vi "Modify Data format to R2_filled+split.vi"(6 "Current set number in one current mode":i32=48, 7 "Scan number":i32=10, 8 "modified error":errorcluster, 9 "modified Data path":path, 10 "original error":errorcluster, 11 "original Data path":path) -> ()   [LabVIEW 2023]
uses:
  <vilib>/Utility/error.llb/DialogType.ctl
panel:
  out "floor(x/y)":i32
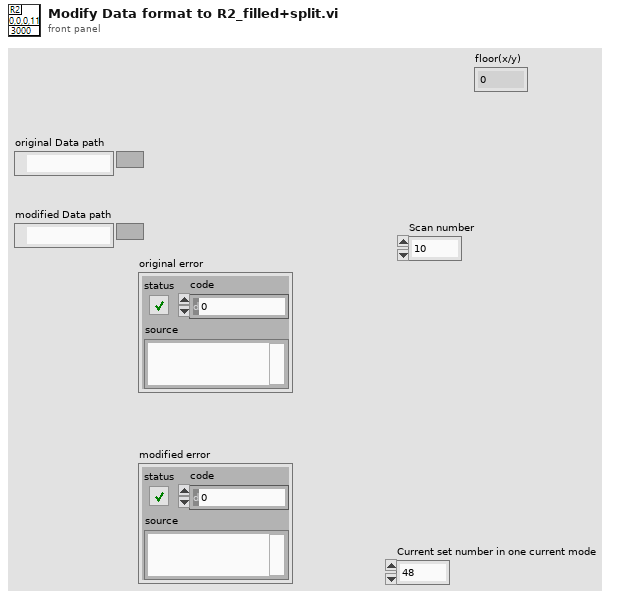
[diagram p1: front panel]
types:
  T1 = enum16{"open", "replace", "create", "open or create", "replace or create", "replace or create with confirmation"}
  T2 = typedef "DialogType.ctl" = u16
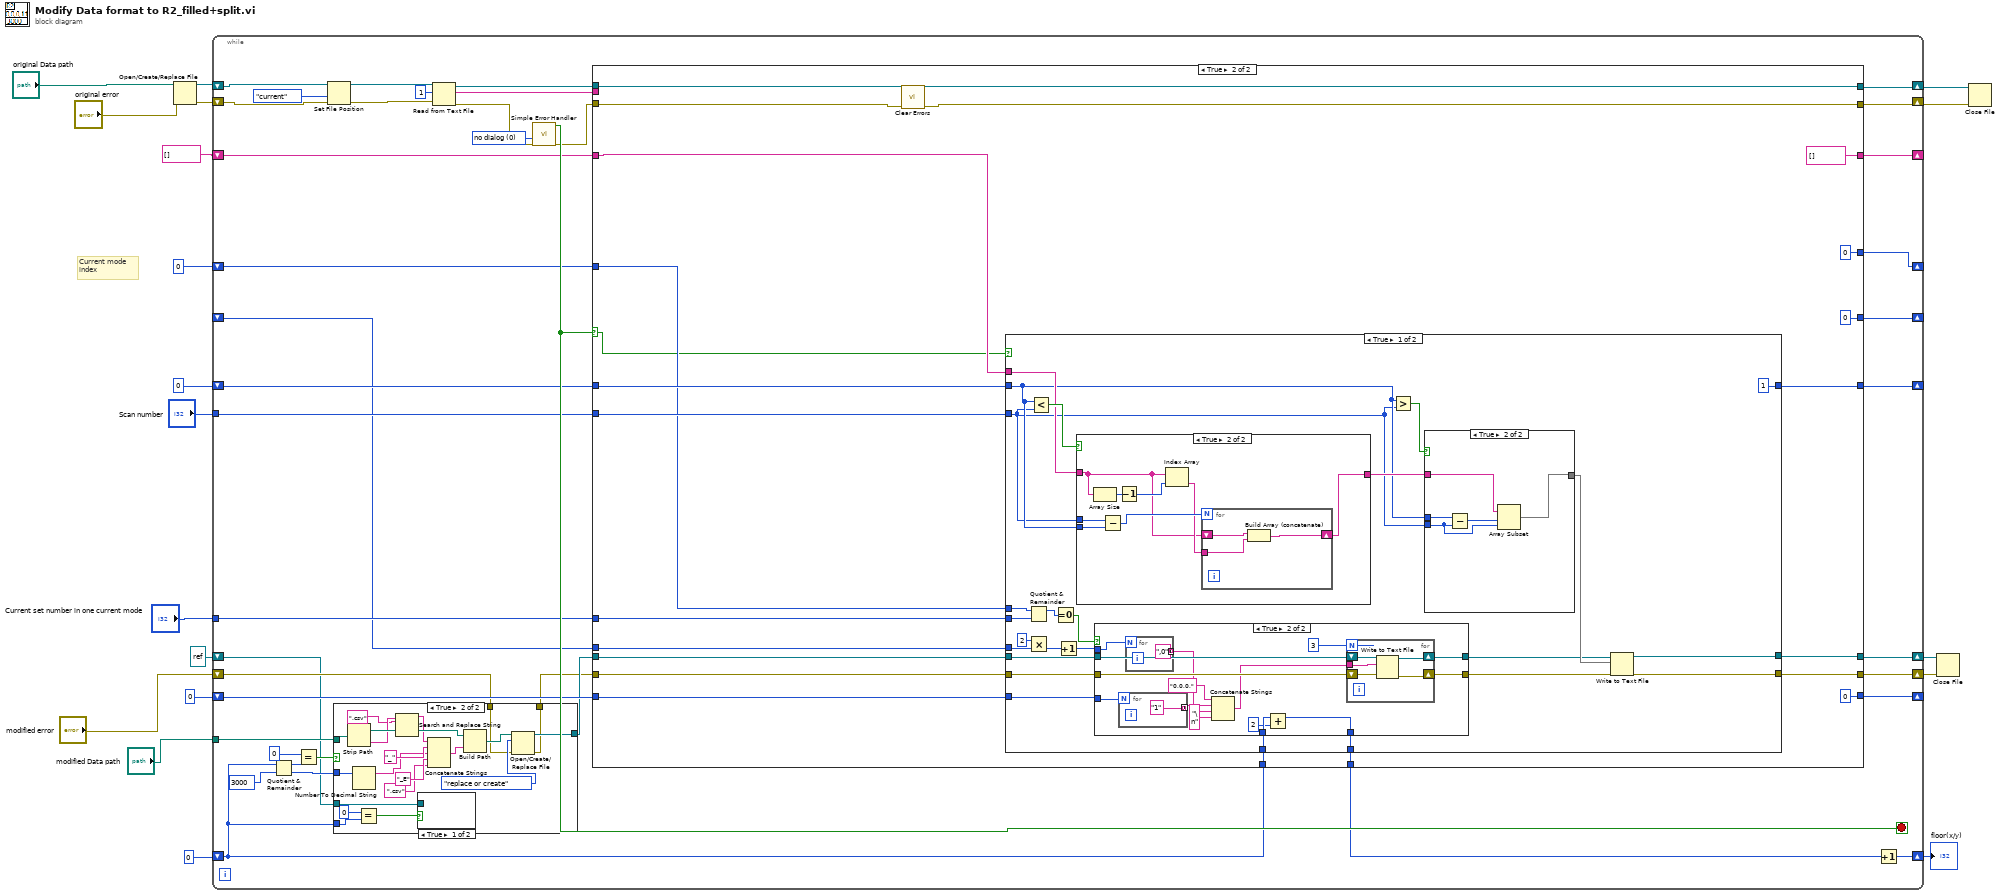
[diagram p0: block diagram]
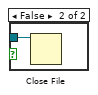
[diagram p3: hidden frame]
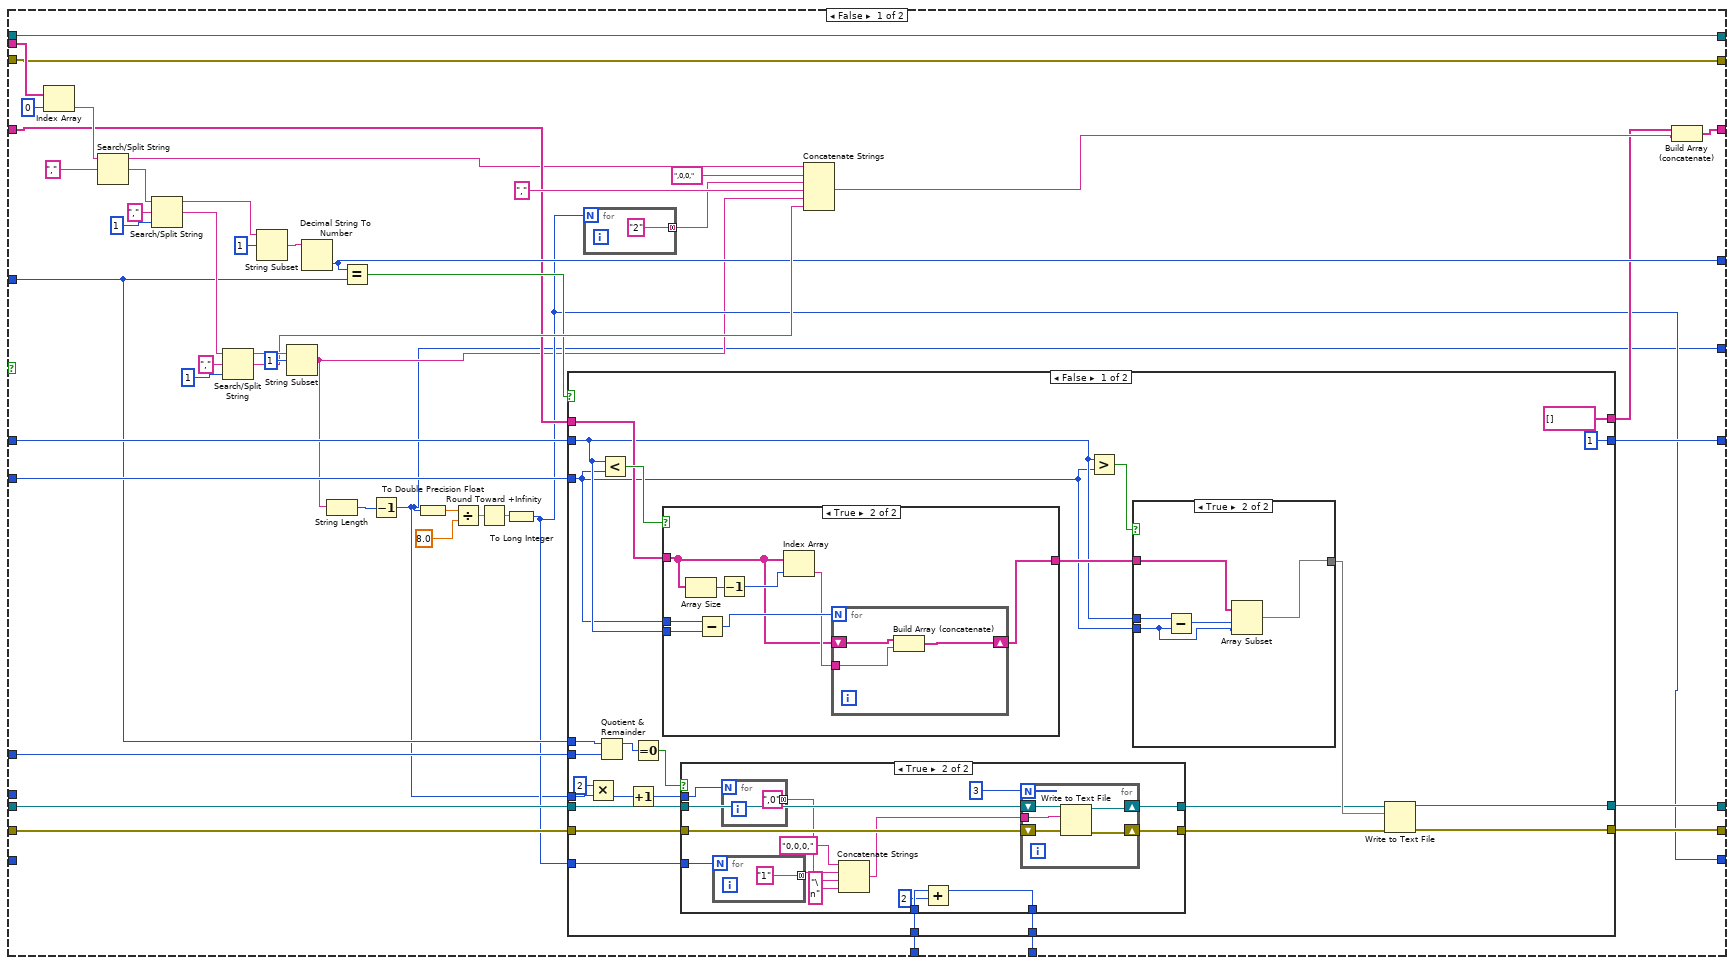
[diagram p4: hidden frame]
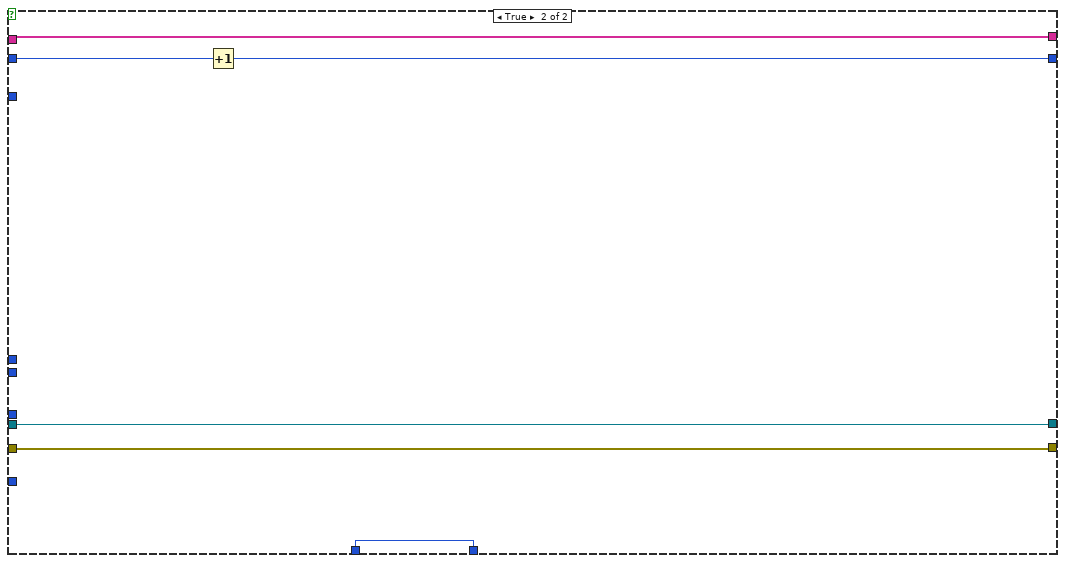
[diagram p8: hidden frame]
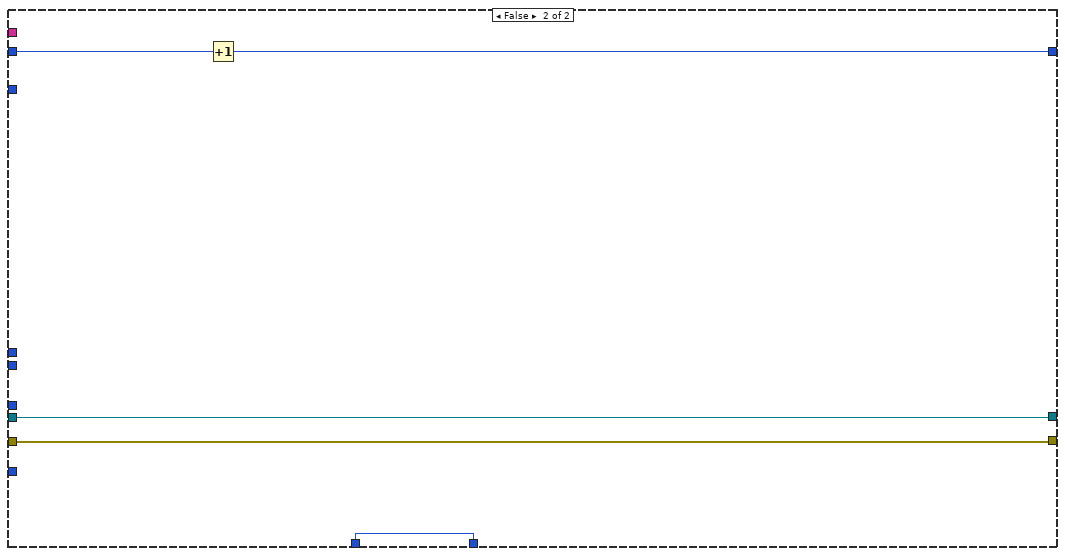
[diagram p12: hidden frame]
diagram:
  # "Current mode\nindex"
  n1 = Open/Create/Replace File(file path (use dialog)="original Data path", error in="original error") -> (refnum out=w17:refnum<file>, error out=w18:errorcluster)  [unwired: 4 in, 1 out]
  n2 = while {
    shift-right: [w52] -> w13
    shift-left: w18 -> [w59]
    shift-right: [w51] -> w19
    shift-left: w17 -> [w50]
    shift-right: [w47] -> w15
    shift-left: refnum<file> refnum ("refnum out") -> [w26]
    shift-right: [w46] -> w14
    shift-left: "modified error" -> [w29]
    shift-right: [w35] -> _
    shift-left: string[] [] ("element") -> [w44]
    shift-right: [w40] -> _
    shift-left: 0 ("number") -> [w43]
    shift-right: [w41] -> _
    shift-left: 0 ("number") -> [w42]
    tunnel: "Scan number" -> [w39]
    tunnel: "Current set number in one current mode" -> [w38]
    shift-right: [w37] -> _
    shift-left: 0 ("32bit integer") -> [w36]
    tunnel: "modified Data path" -> [w27]
    shift-right: [w25] -> w1
    shift-left: 0 ("floor(x/y)") -> [w24]
    shift-right: [w22] -> _
    shift-left: _ -> [w21]
    stop <- w56 stop-if-true
    w57 = T2 0 items=["no dialog", "OK message", "continue or stop message", "OK message + warnings", "continue/stop + warnings"] ("type of dialog (OK msg:1)")
    n3 = Quotient & Remainder(x=w24, y=3000) -> (x-y*floor(x/y)=w34:i32, floor(x/y)=w31:i32)
    n4 = Equal?(x=0, y=w34) -> (x = y?=w32:bool)
    n5 = Set File Position(refnum=w50, from (0:start)=enum16{"start", "end", "current"}."current", error in=w59) -> (refnum out=w49:refnum<file>, error out=w48:errorcluster)  [unwired: 1 in]
    n6 = case shown="True" w32 {
      tunnel: w27 -> [_ w76]
      tunnel: w31 -> [_ w78]
      tunnel: [w61 w73] -> w30
      tunnel: w29 -> [w62 w72]
      tunnel: [w62 w71] -> w28
      tunnel: w26 -> [w61 w70]
      tunnel: w24 -> [_ w68]
      frame False {
      }
      frame True {
        n7 = Strip Path(path=w76) -> (stripped path=w82:path, name=w64:string)
        n8 = Number To Decimal String(number=w78) -> (decimal integer string=w77:string)  [unwired: 1 in]
        n9 = Equal?(x=0, y=w68) -> (x = y?=w66:bool)
        n10 = Search and Replace String(input string=w64, search string=".csv") -> (result string=w65:string)  [unwired: 6 in, 3 out]
        n11 = case shown="True" w66 {
          tunnel: w70 -> [_ w83]
          frame True {
          }
          frame False {
            n12 = Close File(refnum=w83) -> ()  [unwired: 1 in, 2 out]
          }
        }
        n13 = Concatenate Strings(w65, "_" ("string"), w77, "_E" ("string"), ".csv" ("string")) -> (w81:string)
        n14 = Build Path(base path=w82, name or relative path=w81) -> (appended path=w74:path)
        n15 = Open/Create/Replace File(file path (use dialog)=w74, error in=w72, operation (0:open)=T1."replace or create") -> (refnum out=w73:refnum<file>, error out=w71:errorcluster)  [unwired: 3 in, 1 out]
      }
    }
    n16 = Read from Text File(file (use dialog)=w49, count=1, error in=w48) -> (refnum out=w54:refnum<file>, text=w55:string[], error out=w53:errorcluster)  [unwired: 1 in, 1 out]
    n17 = call <vilib>:"Simple Error Handler.vi"("type of dialog (OK msg:1)"=w57, "error in (no error)"=w53) -> ("error?"=w56:bool, "error out"=w45:errorcluster)  [unwired: 3 in, 3 out]
    n18 = case shown="True" w56 {
      selector: w56 -> [_ w215]
      tunnel: w55 -> [w125 _]
      tunnel: w54 -> [w123 w228]
      tunnel: w45 -> [w122 w217]
      tunnel: [w123 w228] -> w51
      tunnel: [w122 w216] -> w52
      tunnel: w30 -> [w103 w223]
      tunnel: w28 -> [w102 w222]
      tunnel: [w101 w221] -> w47
      tunnel: [w100 w220] -> w46
      tunnel: w44 -> [w105 w224]
      tunnel: w43 -> [w99 w219]
      tunnel: w42 -> [w110 w227]
      tunnel: [w109 w226] -> w41
      tunnel: [w108 0] -> w40
      tunnel: w39 -> [w106 w225]
      tunnel: w38 -> [w98 w218]
      tunnel: [w90 0] -> w37
      tunnel: w36 -> [_ w212]
      tunnel: [w89 string[] [] ("element")] -> w35
      tunnel: w24 -> [w86 w207]
      tunnel: [w85 w208] -> w23
      tunnel: [w84 0] -> w22
      tunnel: w21 -> [_ w209]
      frame False {
        n19 = Index Array(array=w125, index=0) -> (element=w121:string)
        n20 = Search/Split String(string=w121, search string/char (-)=",") -> (substring before match=w93:string, match + rest of string=w130:string)  [unwired: 1 in, 1 out]
        n21 = Search/Split String(string=w130, search string/char (-)=",", offset (0)=1) -> (substring before match=w113:string, match + rest of string=w118:string)  [unwired: 1 out]
        n22 = Search/Split String(string=w118, search string/char (-)=",", offset (0)=1) -> (substring before match=w117:string, match + rest of string=w115:string)  [unwired: 1 out]
        n23 = String Subset(string=w113, offset (0)=1) -> (substring=w112:string)  [unwired: 1 in]
        n24 = String Subset(string=w117, offset (0)=1) -> (substring=w88:string)  [unwired: 1 in]
        n25 = Decimal String To Number(string=w112) -> (number=w108:i32)  [unwired: 2 in, 1 out]
        n26 = String Length(string=w88) -> (length=w87:i32)
        n27 = Equal?(x=w108, y=w99) -> (x = y?=w111:bool)
        n28 = Decrement(x=w87) -> (x-1=w84:i32)
        n29 = To Double Precision Float(number=w84) -> (double precision float=w96:dbl)
        n30 = Divide(x=w96, y=8.0) -> (x/y=w97:dbl)
        n31 = Round Toward +Infinity(x=w97) -> (ceil(x): smallest int >= x=w94:dbl)
        n32 = To Long Integer(number=w94) -> (32bit integer=w90:i32)
        n33 = case shown="False" w111 {
          tunnel: [1 w205] -> w109
          tunnel: w110 -> [w151 w206]
          tunnel: w106 -> [w150 _]
          tunnel: w105 -> [w154 w204]
          tunnel: [string[] [] ("element") w204] -> w104
          tunnel: w103 -> [w142 w203]
          tunnel: w102 -> [w141 w202]
          tunnel: [w148 w203] -> w101
          tunnel: [w147 w202] -> w100
          tunnel: w99 -> [w146 _]
          tunnel: w98 -> [w145 _]
          tunnel: w90 -> [w138 _]
          tunnel: w84 -> [w137 _]
          tunnel: w86 -> [w133 w201]
          tunnel: [w132 w201] -> w85
          frame False {
            n34 = Multiply(x=2, y=w137) -> (x*y=w136:i32)
            n35 = Quotient & Remainder(x=w146, y=w145) -> (x-y*floor(x/y)=w144:i32)  [unwired: 1 out]
            n36 = Less?(x=w151, y=w150) -> (x < y?=w155:bool)
            n37 = Increment(x=w136) -> (x+1=w134:i32)
            n38 = Equal To 0?(x=w144) -> (x = 0?=w143:bool)
            n39 = case shown="True" w155 {
              tunnel: w154 -> [w189 w191]
              tunnel: w150 -> [_ w195]
              tunnel: w151 -> [_ w194]
              tunnel: [w189 w190] -> w152
              frame False {
              }
              frame True {
                n40 = Array Size(array=w191) -> (size(s)=w197:i32)
                n41 = Subtract(x=w195, y=w194) -> (x-y=w193:i32)
                n42 = Decrement(x=w197) -> (x-1=w196:i32)
                n43 = Index Array(array=w191, index=w196) -> (element=w192:string)
                n44 = for {
                  N: w193 -> [_]
                  tunnel: w192 -> [w198]
                  shift-right: [w199] -> w190
                  shift-left: w191 -> [w200]
                  n45 = Build Array (concatenate)(w200, w198) -> (w199:string[])
                }
              }
            }
            n46 = case shown="True" w143 {
              tunnel: w142 -> [w160 w172]
              tunnel: w141 -> [w159 w171]
              tunnel: [w160 w169] -> w140
              tunnel: [w159 w168] -> w139
              tunnel: w138 -> [_ w167]
              tunnel: w134 -> [_ w166]
              tunnel: w133 -> [w158 w163]
              tunnel: [w158 w162] -> w132
              frame False {
              }
              frame True {
                n47 = for {
                  N: w167 -> [_]
                  tunnel: ["1" ("search string/char (-)")] -> w174 mode=concatenating
                }
                n48 = for {
                  N: w166 -> [_]
                  tunnel: [",0" ("search string/char (-)")] -> w164 mode=concatenating
                }
                n49 = Concatenate Strings("0,0,0," ("string"), w174, w164, "\n" ("string")) -> (w170:string)
                n50 = Add(x=w163, y=2) -> (x+y=w162:i32)
                n51 = for {
                  N: 3 -> [_]
                  shift-right: [w179] -> w169
                  shift-left: w172 -> [w182]
                  tunnel: w170 -> [w180]
                  shift-right: [w178] -> w168
                  shift-left: w171 -> [w181]
                  n52 = Write to Text File(file (use dialog)=w182, text=w180, error in=w181) -> (refnum out=w179:refnum<file>, error out=w178:errorcluster)  [unwired: 1 in, 1 out]
                }
              }
            }
            n53 = Greater?(x=w151, y=w150) -> (0:w153:bool)
            n54 = case shown="True" w153 {
              tunnel: w152 -> [w183 w187]
              tunnel: w151 -> [_ w188]
              tunnel: w150 -> [_ w185]
              tunnel: [w183 w184] -> w149
              frame False {
              }
              frame True {
                n55 = Subtract(x=w188, y=w185) -> (x-y=w186:i32)
                n56 = Array Subset(array=w187, index=w186, length=w185) -> (w184:string[])
              }
            }
            n57 = Write to Text File(file (use dialog)=w140, text=w149, error in=w139) -> (refnum out=w148:refnum<file>, error out=w147:errorcluster)  [unwired: 1 in, 1 out]
          }
          frame True {
            n58 = Increment(x=w206) -> (x+1=w205:i32)
          }
        }
        n59 = for {
          N: w90 -> [_]
          tunnel: ["2" ("search string/char (-)")] -> w91 mode=concatenating
        }
        n60 = Concatenate Strings(w93, ",0,0," ("string"), w91, "," ("string"), w88, w115) -> (w107:string)
        n61 = Build Array (concatenate)(w104, w107) -> (w89:string[])
      }
      frame True {
        n62 = call <vilib>:"Clear Errors.vi"("error in (no error)"=w217) -> ("error out"=w216:errorcluster)  [unwired: 5 in, 1 out]
        n63 = case shown="True" w215 {
          tunnel: [1 w300] -> w226
          tunnel: w227 -> [w248 w301]
          tunnel: w225 -> [w247 _]
          tunnel: w224 -> [w251 _]
          tunnel: w223 -> [w236 w299]
          tunnel: w222 -> [w235 w298]
          tunnel: [w245 w299] -> w221
          tunnel: [w244 w298] -> w220
          tunnel: w219 -> [w243 _]
          tunnel: w218 -> [w242 _]
          tunnel: w212 -> [w234 _]
          tunnel: w209 -> [w231 _]
          tunnel: [w230 w297] -> w208
          tunnel: w207 -> [w229 w297]
          frame True {
            n64 = Quotient & Remainder(x=w243, y=w242) -> (x-y*floor(x/y)=w241:i32)  [unwired: 1 out]
            n65 = Multiply(x=2, y=w231) -> (x*y=w239:i32)
            n66 = Less?(x=w248, y=w247) -> (x < y?=w252:bool)
            n67 = Equal To 0?(x=w241) -> (x = 0?=w237:bool)
            n68 = Increment(x=w239) -> (x+1=w240:i32)
            n69 = case shown="True" w252 {
              tunnel: w251 -> [w285 w287]
              tunnel: w247 -> [_ w291]
              tunnel: w248 -> [_ w290]
              tunnel: [w285 w286] -> w249
              frame False {
              }
              frame True {
                n70 = Array Size(array=w287) -> (size(s)=w293:i32)
                n71 = Subtract(x=w291, y=w290) -> (x-y=w289:i32)
                n72 = Decrement(x=w293) -> (x-1=w292:i32)
                n73 = Index Array(array=w287, index=w292) -> (element=w288:string)
                n74 = for {
                  N: w289 -> [_]
                  tunnel: w288 -> [w294]
                  shift-right: [w295] -> w286
                  shift-left: w287 -> [w296]
                  n75 = Build Array (concatenate)(w296, w294) -> (w295:string[])
                }
              }
            }
            n76 = case shown="True" w237 {
              tunnel: w236 -> [w256 w268]
              tunnel: w235 -> [w255 w267]
              tunnel: [w256 w265] -> w233
              tunnel: [w255 w264] -> w232
              tunnel: w234 -> [_ w263]
              tunnel: w240 -> [_ w262]
              tunnel: [w254 w258] -> w230
              tunnel: w229 -> [w254 w259]
              frame False {
              }
              frame True {
                n77 = for {
                  N: w263 -> [_]
                  tunnel: ["1" ("search string/char (-)")] -> w270 mode=concatenating
                }
                n78 = for {
                  N: w262 -> [_]
                  tunnel: [",0" ("search string/char (-)")] -> w260 mode=concatenating
                }
                n79 = Concatenate Strings("0,0,0," ("string"), w270, w260, "\n" ("string")) -> (w266:string)
                n80 = Add(x=w259, y=2) -> (x+y=w258:i32)
                n81 = for {
                  N: 3 -> [_]
                  shift-right: [w275] -> w265
                  shift-left: w268 -> [w278]
                  tunnel: w266 -> [w276]
                  shift-right: [w274] -> w264
                  shift-left: w267 -> [w277]
                  n82 = Write to Text File(file (use dialog)=w278, text=w276, error in=w277) -> (refnum out=w275:refnum<file>, error out=w274:errorcluster)  [unwired: 1 in, 1 out]
                }
              }
            }
            n83 = Greater?(x=w248, y=w247) -> (0:w250:bool)
            n84 = case shown="True" w250 {
              tunnel: w249 -> [w279 w283]
              tunnel: w248 -> [_ w284]
              tunnel: w247 -> [_ w281]
              tunnel: [w279 w280] -> w246
              frame False {
              }
              frame True {
                n85 = Subtract(x=w284, y=w281) -> (x-y=w282:i32)
                n86 = Array Subset(array=w283, index=w282, length=w281) -> (w280:string[])
              }
            }
            n87 = Write to Text File(file (use dialog)=w233, text=w246, error in=w232) -> (refnum out=w245:refnum<file>, error out=w244:errorcluster)  [unwired: 1 in, 1 out]
          }
          frame False {
            n88 = Increment(x=w301) -> (x+1=w300:i32)
          }
        }
      }
    }
    n89 = Increment(x=w23) -> (x+1=w25:i32)
  }
  "floor(x/y)" <- w1
  n90 = Close File(refnum=w15, error in=w14) -> ()  [unwired: 2 out]
  n91 = Close File(refnum=w19, error in=w13) -> ()  [unwired: 2 out]
